vi "main.vi"(8 "error in (no error)":errorcluster, 11 "interface":T1) -> (0 "error out":errorcluster)   [LabVIEW 2015, in "lv-interface-sub-re.lvlib"]
uses:
  lv-interface-sub-re.lvlib
  lv-interface-sub-common/_controls/interface_selection.ctl
  private/_controls/hmi_references.ctl
  private/_controls/hmi_states.ctl
  private/_controls/event_common.ctl
  private/_controls/event_common_command.ctl
  private/_controls/event_interface.ctl
  private/_controls/event_interface_command.ctl
  private/_controls/menu_selection.ctl
  lv-interface-sub-common/lv-interface-sub-common.lvlib
panel:
  out "random_number":dbl
  out "source":string
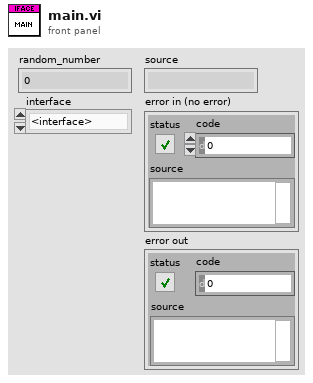
[diagram p1: front panel]
types:
  T1 = typedef "lv-interface-sub-common.lvlib/interface_selection.ctl" = enum16{"<interface>", "sub_interface_1", "sub_interface_2", "<null>"}
  T2 = typedef "lv-interface-sub-re.lvlib/hmi_references.ctl" = cluster{"vi_reference":refnum<vi>}
  T3 = typedef "lv-interface-sub-re.lvlib/event_interface.ctl" = cluster{"command":T4, "data":variant}
  T4 = typedef "lv-interface-sub-re.lvlib/event_interface_command.ctl" = enum16{"<event_interface_cmd>", "defer_panel_updates", "focus", "unfocus", "undefer_panel_updates", "<null>"}
  T5 = typedef "lv-interface-sub-re.lvlib/event_common.ctl" = cluster{"command":T6, "data":variant}
  T6 = typedef "lv-interface-sub-re.lvlib/event_common_command.ctl" = enum16{"<event_common_cmd>", "die", "<null>"}
  T7 = typedef "lv-interface-sub-re.lvlib/hmi_states.ctl" = enum16{"<hmi_states>", "initialize", "checkui", "updateui", "shutdown", "<null>"}
  T8 = typedef "lv-interface-sub-re.lvlib/menu_selection.ctl" = enum16{"<menu>", "file_exit", "help_about", "<null>"}
  T9 = typedef "interface_dom_nre.lvlib/interface_selection.ctl" = enum16{"<interface>", "sub_interface_1", "sub_interface_2", "<null>"}
  T10 = typedef "interface_sub_common.lvlib/event_to_sub_command.ctl" = enum16{"<to_sub_cmd>", "die", "focus", "unfocus", "<null>"}
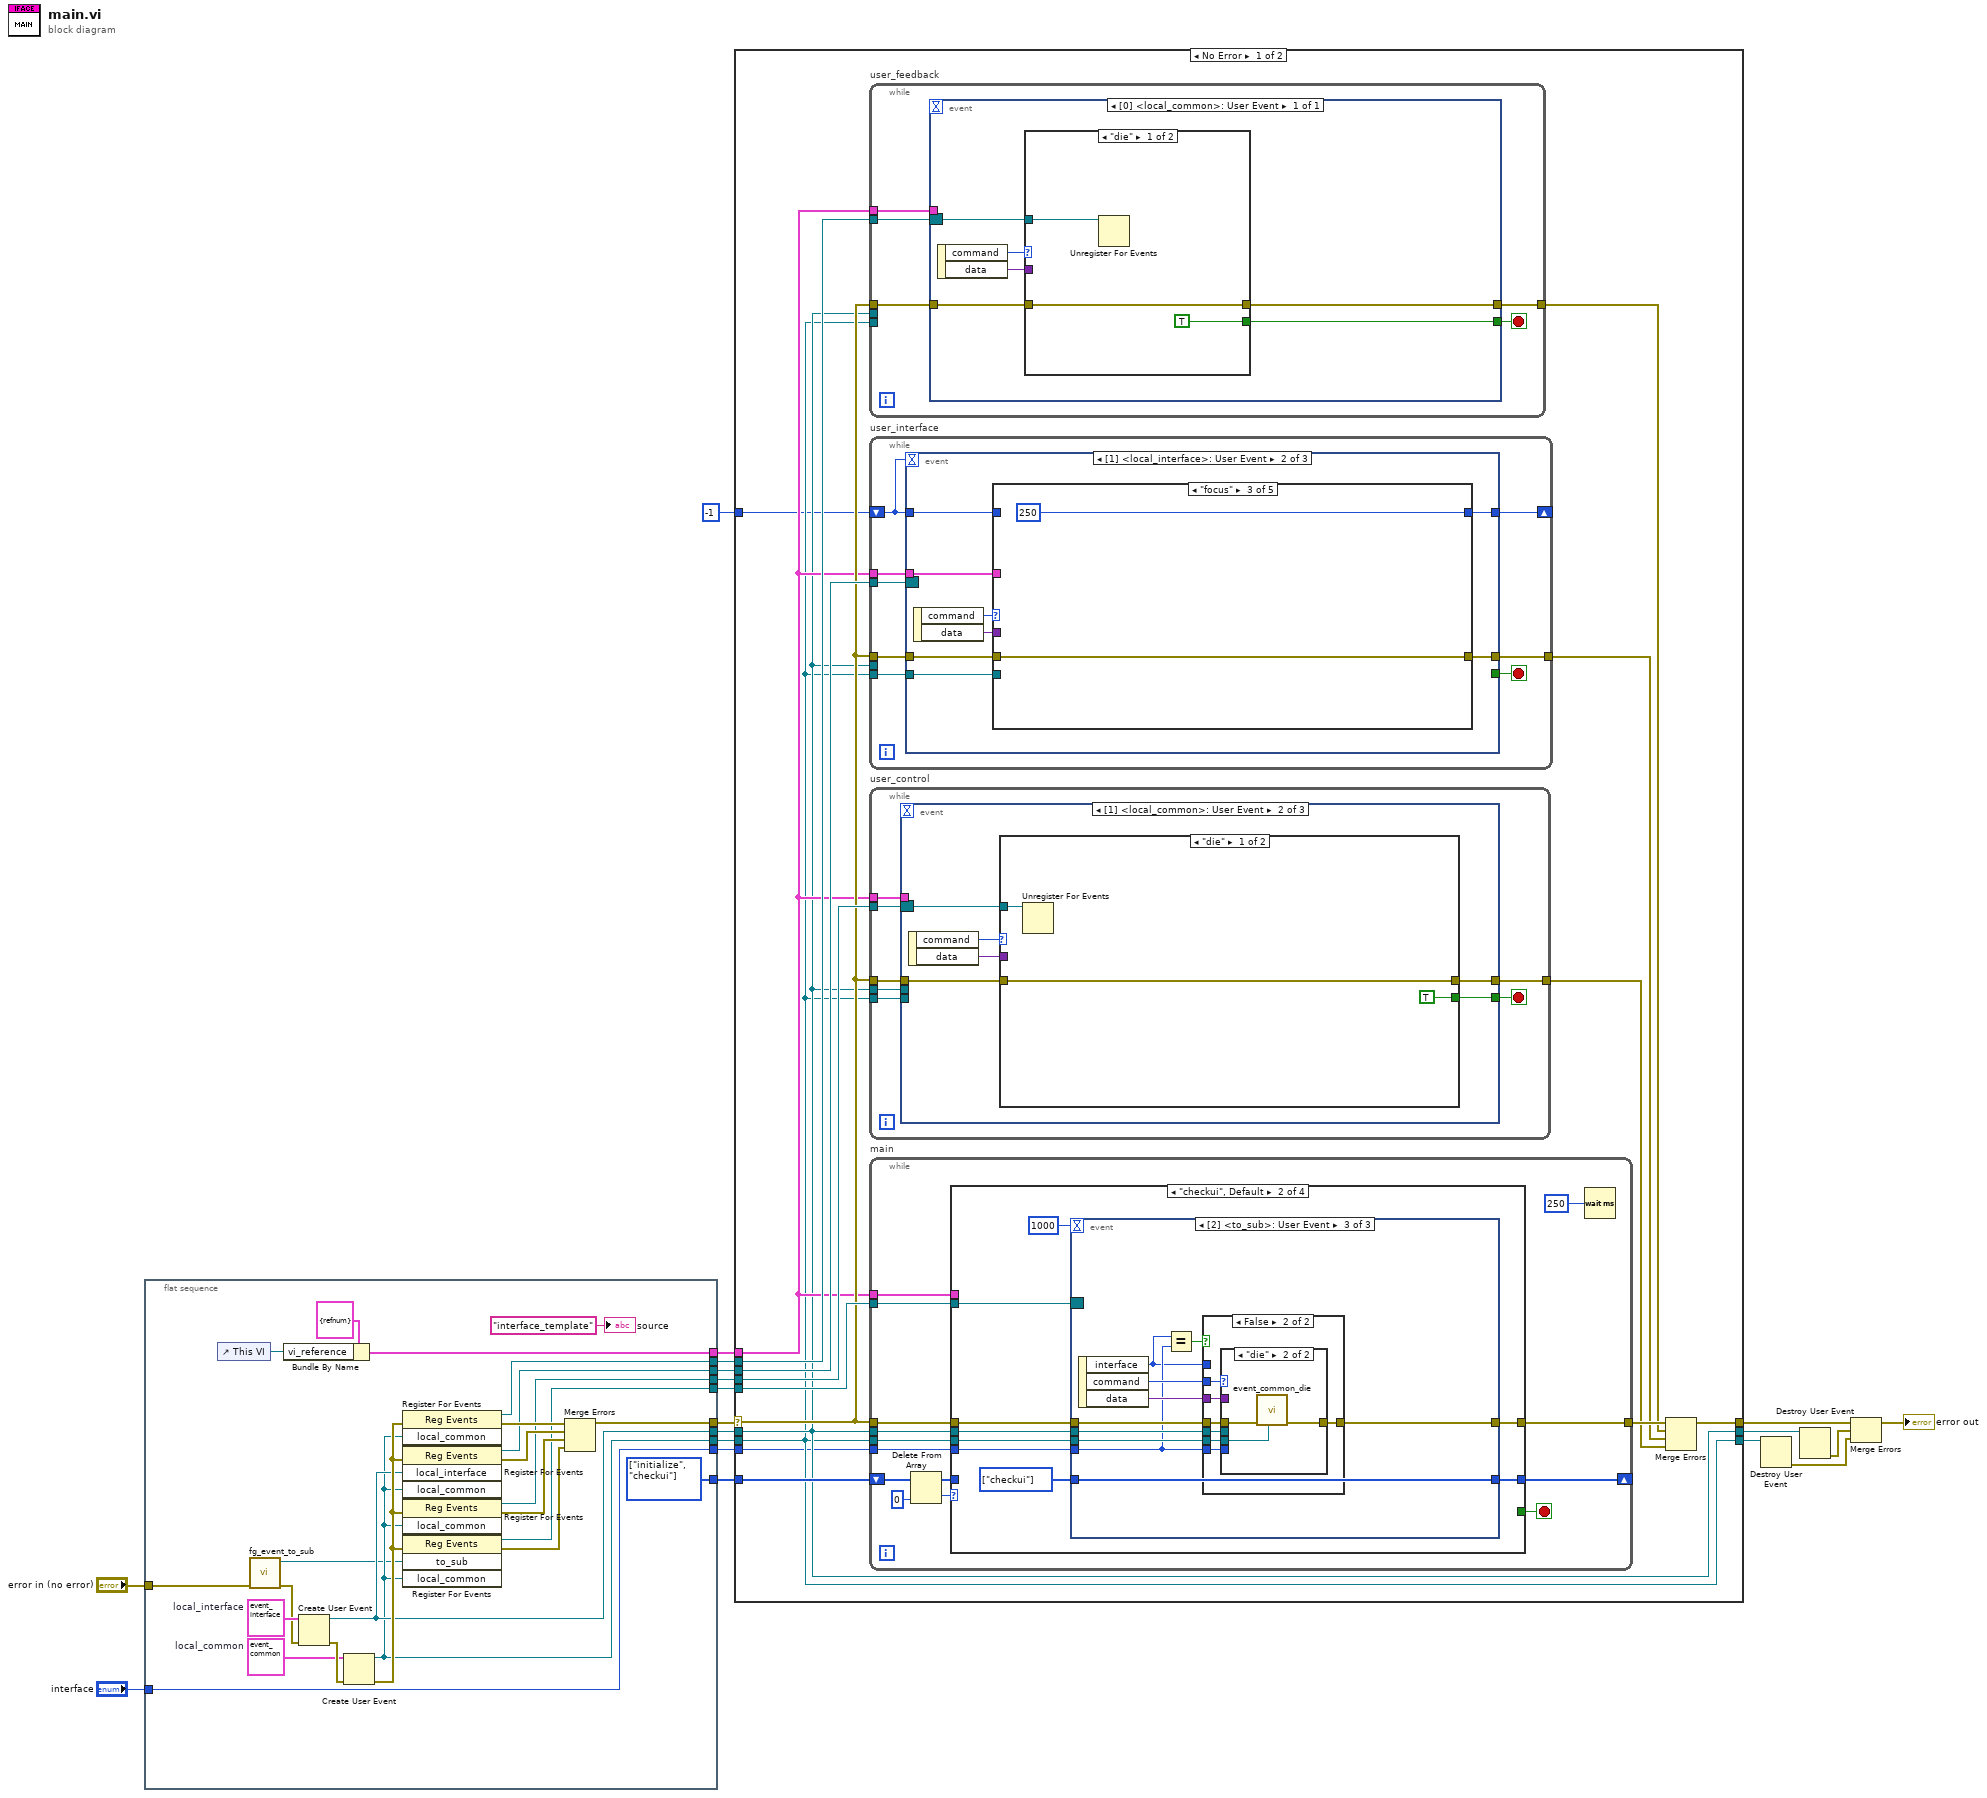
[diagram p0: block diagram]
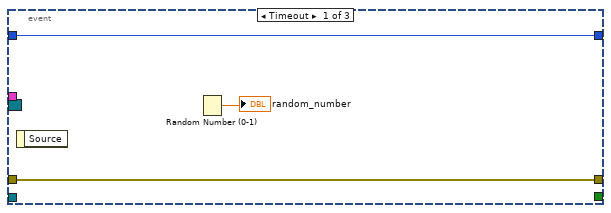
[diagram p3: hidden frame]
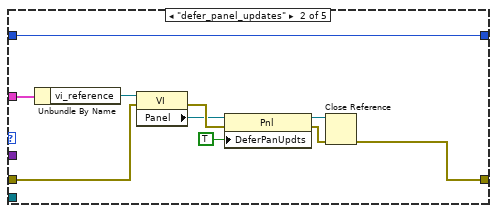
[diagram p5: hidden frame]
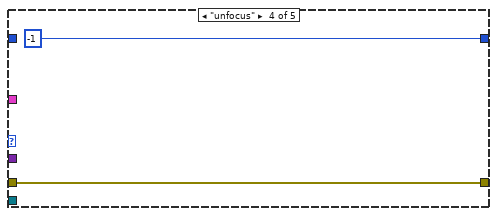
[diagram p6: hidden frame]
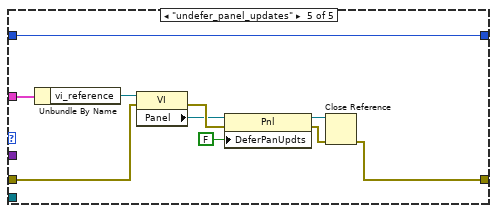
[diagram p7: hidden frame]
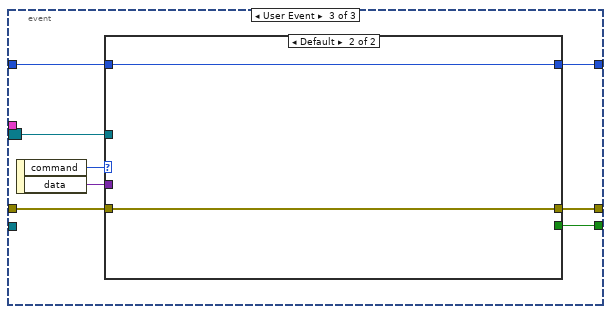
[diagram p8: hidden frame]
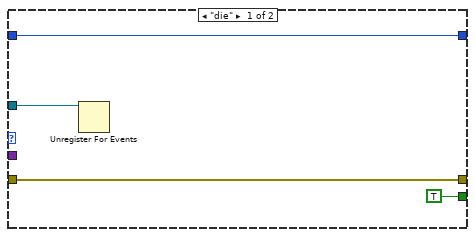
[diagram p9: hidden frame]
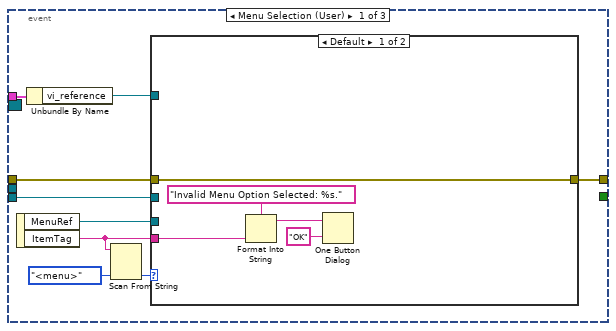
[diagram p10: hidden frame]
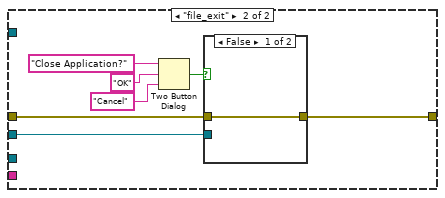
[diagram p11: hidden frame]
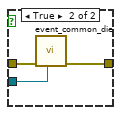
[diagram p12: hidden frame]
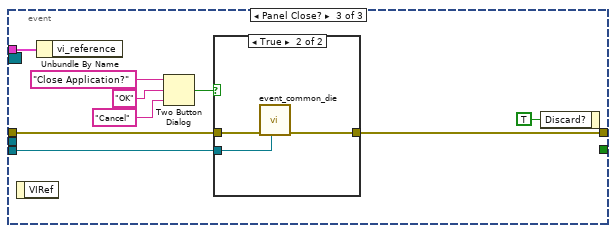
[diagram p14: hidden frame]
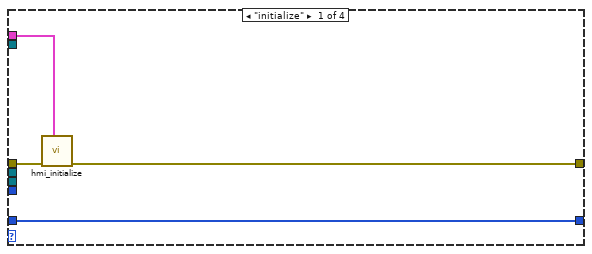
[diagram p16: hidden frame]
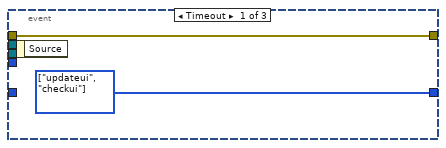
[diagram p17: hidden frame]
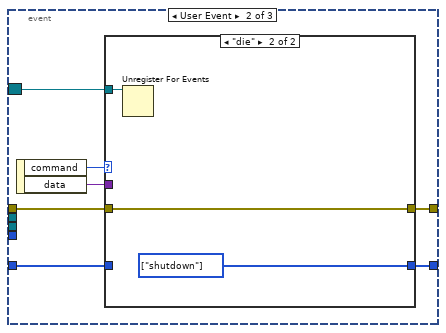
[diagram p18: hidden frame]
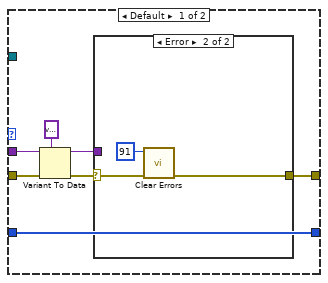
[diagram p19: hidden frame]
diagram:
  n1 = flat-sequence {
    tunnel: [w35] -> w19
    tunnel: [w34] -> w18
    tunnel: [w38] -> w17
    tunnel: "error in (no error)" -> [w22]
    tunnel: [w33] -> w15
    tunnel: [w32] -> w14
    tunnel: [w30] -> w13
    tunnel: [w24] -> w11
    tunnel: [w27] -> w12
    tunnel: [w25] -> w5
    tunnel: "interface" -> [w20]
    tunnel: [w20] -> w1
    frame #0 {
      w28 = T3 {"command"=enum."<event_interface_cmd>", "data"=variant}  # local_interface
      w29 = T5 {"command"=enum."<event_common_cmd>", "data"=variant}  # local_common
      w38 = T7[] [enum."initialize", enum."checkui"] items=["<hmi_states>", "initialize", "checkui", "updateui", "shutdown", "<null>"]
      n2 = control-ref of="This VI"() -> (w31:refnum<vi>)
      n3 = call "fg_event_to_sub.vi"("error in (no error)"=w22) -> ("error out"=w21:errorcluster, "to_sub"=w23:refnum<user-event>)  [unwired: 8 in, 1 out]
      n4 = Bundle By Name(cluster=T2 {"vi_reference"=refnum}, "vi_reference"=w31) -> (w30:T2)
      n5 = Create User Event(user event datatype=w28, error in=w21) -> (user event=w27:refnum<user-event>, error out=w42:errorcluster)
      n6 = Create User Event(user event datatype=w29, error in=w42) -> (user event=w24:refnum<user-event>, error out=w41:errorcluster)
      n7 = register-events(error in=w41, w24) -> (reference out=w25:refnum<event-registration>, error out=w43:errorcluster)  [unwired: 1 in]
      n8 = register-events(error in=w41, w27, w24) -> (reference out=w32:refnum<event-registration>, error out=w40:errorcluster)  [unwired: 1 in]
      n9 = register-events(error in=w41, w24) -> (reference out=w34:refnum<event-registration>, error out=w37:errorcluster)  [unwired: 1 in]
      n10 = register-events(error in=w41, w23, w24) -> (reference out=w33:refnum<event-registration>, error out=w36:errorcluster)  [unwired: 1 in]
      n11 = Merge Errors(w43, w40, w37, w36) -> (w35:errorcluster)
      "source" <- "interface_template" ("Source")
    }
  }
  n12 = case shown="No Error" w19 {
    selector: w19 -> [w50 w290]
    tunnel: w18 -> [w53 w286]
    tunnel: w17 -> [w55 _]
    tunnel: [w51 w290] -> w8
    tunnel: w15 -> [w54 w285]
    tunnel: w14 -> [w52 w287]
    tunnel: w13 -> [w49 _]
    tunnel: w12 -> [w48 w289]
    tunnel: w11 -> [w47 w288]
    tunnel: [w48 w289] -> w9
    tunnel: [w47 w288] -> w10
    tunnel: w5 -> [w59 w284]
    tunnel: -1 -> [w45 _]
    tunnel: w1 -> [w44 _]
    frame No Error {
      n13 = while "user_feedback" {
        tunnel: [w64] -> w46
        tunnel: w50 -> [w63]
        tunnel: w59 -> [w62]
        tunnel: w49 -> [w61]
        tunnel: w48 -> [_]
        tunnel: w47 -> [_]
        stop <- w60 stop-if-true
        n14 = event shown="[0] <local_common>: User Event" {
          selector: w62 -> [w70]
          dyn-events: _ -> [_]
          timeout: _ -> [_]
          tunnel: [w67] -> w64
          tunnel: w63 -> [w68]
          tunnel: w61 -> [_]
          tunnel: [w66] -> w60
          event User Event {
            n15 = event-data() -> ("command"=w69:T6, "data"=w65:variant)  [unwired: 1 in]
            n16 = case shown="\"die\"" w69 {
              tunnel: w68 -> [w72 w74]
              tunnel: [w72 w74] -> w67
              tunnel: [TRUE _] -> w66
              tunnel: w70 -> [w71 _]
              tunnel: w65 -> [_ _]
              frame "die" {
                n17 = Unregister For Events(event registration refnum=w71) -> ()  [unwired: 1 in, 1 out]
              }
              frame Default {
              }
            }
          }
        }
      }
      n18 = while "user_interface" {
        tunnel: w50 -> [w82]
        tunnel: [w80] -> w56
        tunnel: w52 -> [w79]
        tunnel: w48 -> [_]
        tunnel: w47 -> [w78]
        tunnel: w49 -> [w77]
        shift-right: [w76] -> _
        shift-left: w45 -> [w75]
        stop <- w81 stop-if-true
        n19 = event shown="[1] <local_interface>: User Event" {
          selector: w79 -> [_ _ w123]
          dyn-events: _ -> [_ _ _]
          timeout: w75 -> [_ _ _]
          tunnel: w82 -> [w83 w91 w126]
          tunnel: [w83 w90 w125] -> w80
          tunnel: [_ _ w124] -> w81
          tunnel: w78 -> [_ w89 _]
          tunnel: w77 -> [_ w88 _]
          tunnel: w75 -> [w85 w87 w121]
          tunnel: [w85 w86 w120] -> w76
          event Timeout {
            n20 = event-data() -> ()  [unwired: 1 in, 1 out]
            n21 = Random Number (0-1)() -> (number: 0 to 1=→"random_number":dbl)
          }
          event User Event {
            n22 = event-data() -> ("command"=w93:T4, "data"=w92:variant)  [unwired: 1 in]
            n23 = case shown="\"focus\"" w93 {
              tunnel: w91 -> [w94 w100 w106 w108 w114]
              tunnel: [w94 w99 w106 w108 w111] -> w90
              tunnel: w92 -> [_ _ _ _ _]
              tunnel: w89 -> [_ _ _ _ _]
              tunnel: w88 -> [_ w98 _ _ w113]
              tunnel: w87 -> [w95 w96 _ _ w110]
              tunnel: [w95 w96 250 -1 w110] -> w86
              frame Default {
              }
              frame "defer_panel_updates" {
                n24 = Unbundle By Name(w98) -> ("vi_reference"=w97:refnum<vi>)
                n25 = property class="VI"(reference=w97, error in=w100) -> (error out=w105:errorcluster, "Panel"=w101:refnum<vi>)  [unwired: 1 out]
                n26 = property class="Pnl"(reference=w101, error in=w105, "DeferPanUpdts"=TRUE ("Defer Panel Updates")) -> (reference out=w103:refnum<vi>, error out=w102:errorcluster)
                n27 = Close Reference(reference=w103, error in (no error)=w102) -> (error out=w99:errorcluster)
              }
              frame "focus" {
              }
              frame "unfocus" {
              }
              frame "undefer_panel_updates" {
                n28 = Unbundle By Name(w113) -> ("vi_reference"=w112:refnum<vi>)
                n29 = property class="VI"(reference=w112, error in=w114) -> (error out=w119:errorcluster, "Panel"=w115:refnum<vi>)  [unwired: 1 out]
                n30 = property class="Pnl"(reference=w115, error in=w119, "DeferPanUpdts"=FALSE ("Defer Panel Updates")) -> (reference out=w117:refnum<vi>, error out=w116:errorcluster)
                n31 = Close Reference(reference=w117, error in (no error)=w116) -> (error out=w111:errorcluster)
              }
            }
          }
          event User Event {
            n32 = event-data() -> ("command"=w127:T6, "data"=w122:variant)  [unwired: 1 in]
            n33 = case shown="Default" w127 {
              tunnel: w126 -> [w130 w133]
              tunnel: [w130 w133] -> w125
              tunnel: [TRUE _] -> w124
              tunnel: w123 -> [w129 _]
              tunnel: w122 -> [_ _]
              tunnel: w121 -> [w128 w132]
              tunnel: [w128 w132] -> w120
              frame "die" {
                n34 = Unregister For Events(event registration refnum=w129) -> ()  [unwired: 1 in, 1 out]
              }
              frame Default {
              }
            }
          }
        }
      }
      n35 = while "user_control" {
        tunnel: w50 -> [w140]
        tunnel: [w138] -> w57
        tunnel: w53 -> [w137]
        tunnel: w48 -> [w135]
        tunnel: w47 -> [w134]
        tunnel: w49 -> [w136]
        stop <- w139 stop-if-true
        n36 = event shown="[1] <local_common>: User Event" {
          selector: w137 -> [_ w166 _]
          dyn-events: _ -> [_ _ _]
          timeout: _ -> [_ _ _]
          tunnel: w140 -> [w146 w170 w176]
          tunnel: [w144 w169 w183] -> w138
          tunnel: [_ w168 _] -> w139
          tunnel: w136 -> [w143 _ w182]
          tunnel: w135 -> [_ _ _]
          tunnel: w134 -> [w141 _ w181]
          event Menu Selection (User) {
            n37 = event-data() -> ("MenuRef"=w147:refnum<k9>, "ItemTag"=w145:string)  [unwired: 1 in]
            n38 = Unbundle By Name(w143) -> ("vi_reference"=w142:refnum<vi>)
            n39 = Scan From String(input string=w145, default 1=menu_selection."<menu>" ("menu_selection")) -> (output 1=w148:T8)  [unwired: 3 in, 3 out]
            n40 = case shown="Default" w148 {
              tunnel: w147 -> [_ _]
              tunnel: w146 -> [w150 w155]
              tunnel: w145 -> [w154 _]
              tunnel: [w150 w161] -> w144
              tunnel: w142 -> [_ _]
              tunnel: w141 -> [_ w160]
              frame Default {
                n41 = Format Into String(format string="Invalid Menu Option Selected: %s.", w154) -> (resulting string=w152:string)  [unwired: 2 in, 1 out]
                n42 = One Button Dialog(message=w152, button name ("OK")="OK" ("boolean_text_1")) -> ()  [unwired: 1 out]
              }
              frame "file_exit" {
                n43 = Two Button Dialog(message="Close Application?" ("dialog_text"), 1:"Cancel" ("boolean_text_1"), 2:"OK" ("boolean_text_1")) -> (T button?=w156:bool)
                n44 = case shown="False" w156 {
                  tunnel: w155 -> [w162 w165]
                  tunnel: [w162 w164] -> w161
                  tunnel: w160 -> [_ w163]
                  frame False {
                  }
                  frame True {
                    n45 = call "event_common_die.vi"("local_common"=w163, "error in (no error)"=w165) -> ("error out"=w164:errorcluster)  [unwired: 9 in]
                  }
                }
              }
            }
          }
          event User Event {
            n46 = event-data() -> ("command"=w171:T6, "data"=w167:variant)  [unwired: 1 in]
            n47 = case shown="\"die\"" w171 {
              tunnel: w170 -> [w172 w175]
              tunnel: [w172 w175] -> w169
              tunnel: [TRUE _] -> w168
              tunnel: w167 -> [_ _]
              tunnel: w166 -> [w173 _]
              frame "die" {
                n48 = Unregister For Events(event registration refnum=w173) -> ()  [unwired: 1 in, 1 out]
              }
              frame Default {
              }
            }
          }
          event Panel Close? {
            n49 = event-data() -> ()  [unwired: 1 in, 1 out]
            n50 = Unbundle By Name(w182) -> ()  [unwired: 1 out]
            n51 = Two Button Dialog(message="Close Application?" ("dialog_text"), 1:"Cancel" ("boolean_text_1"), 2:"OK" ("boolean_text_1")) -> (T button?=w177:bool)
            n52 = case shown="True" w177 {
              tunnel: w176 -> [w185 w188]
              tunnel: [w185 w187] -> w183
              tunnel: w181 -> [_ w186]
              frame False {
              }
              frame True {
                n53 = call "event_common_die.vi"("local_common"=w186, "error in (no error)"=w188) -> ("error out"=w187:errorcluster)  [unwired: 9 in]
              }
            }
            n54 = event-data("Discard?"=TRUE) -> ()  [unwired: 1 in, 1 out]
          }
        }
      }
      n55 = while "main" {
        shift-right: [w194] -> _
        shift-left: w55 -> [w201]
        tunnel: w54 -> [w195]
        tunnel: w50 -> [w197]
        tunnel: [w193] -> w58
        tunnel: w49 -> [w192]
        tunnel: w47 -> [w191]
        tunnel: w48 -> [w190]
        tunnel: w44 -> [w189]
        stop <- w196 stop-if-true
        n56 = Delete From Array(array=w201, index=0) -> (deleted portion=w199:T7, array with subset deleted=w198:T7[])  [unwired: 1 in]
        n57 = case shown="\"checkui\", Default" w199 {
          tunnel: w198 -> [w206 _ w278 _]
          tunnel: w197 -> [w205 w214 w277 w282]
          tunnel: [_ _ _ TRUE] -> w196
          tunnel: [w203 w213 w277 w281] -> w193
          tunnel: [w206 w212 w278 w280] -> w194
          tunnel: w195 -> [_ w210 _ _]
          tunnel: w192 -> [w204 _ _ w279]
          tunnel: w191 -> [_ w208 _ _]
          tunnel: w190 -> [_ w209 _ _]
          tunnel: w189 -> [_ w207 _ _]
          frame "initialize" {
            n58 = call "hmi_initialize.vi"("hmi_references"=w204, "error in (no error)"=w205) -> ("error out"=w203:errorcluster)  [unwired: 9 in]
          }
          frame "checkui", Default {
            w211 = T7[] [enum."checkui"] items=["<hmi_states>", "initialize", "checkui", "updateui", "shutdown", "<null>"]
            n59 = event shown="[2] <to_sub>: User Event" {
              selector: w210 -> [_ w218 _]
              dyn-events: _ -> [_ _ _]
              timeout: 1000 -> [_ _ _]
              tunnel: w214 -> [w217 w222 w246]
              tunnel: [w217 w219 w245] -> w213
              tunnel: [w216 w220 w242] -> w212
              tunnel: w211 -> [_ w221 w242]
              tunnel: w209 -> [_ _ w244]
              tunnel: w208 -> [_ _ w243]
              tunnel: w207 -> [_ _ w241]
              event Timeout {
                w216 = T7[] [enum."updateui", enum."checkui"] items=["<hmi_states>", "initialize", "checkui", "updateui", "shutdown", "<null>"]
                n60 = event-data() -> ()  [unwired: 1 in, 1 out]
              }
              event User Event {
                n61 = event-data() -> ("command"=w224:T6, "data"=w223:variant)  [unwired: 1 in]
                n62 = case shown="\"die\"" w224 {
                  tunnel: [w231 w238] -> w220
                  tunnel: w221 -> [w231 _]
                  tunnel: w222 -> [w229 w237]
                  tunnel: [w225 w237] -> w219
                  tunnel: w223 -> [w230 _]
                  tunnel: w218 -> [_ w236]
                  frame Default {
                    n63 = Variant To Data(error in=w229, type=variant, Variant=w230) -> (data=w226:variant, error out=w228:errorcluster)
                    n64 = case shown="Error" w228 {
                      selector: w228 -> [w232 w235]
                      tunnel: w226 -> [_ _]
                      tunnel: [w232 w234] -> w225
                      frame No Error {
                      }
                      frame Error {
                        n65 = call <vilib>:"Clear Errors.vi"("error in (no error)"=w235, "specific error code to clear (0: all)"=91) -> ("error out"=w234:errorcluster)  [unwired: 4 in, 1 out]
                      }
                    }
                  }
                  frame "die" {
                    w238 = T7[] [enum."shutdown"] items=["<hmi_states>", "initialize", "checkui", "updateui", "shutdown", "<null>"]
                    n66 = Unregister For Events(event registration refnum=w236) -> ()  [unwired: 1 in, 1 out]
                  }
                }
              }
              event User Event {
                n67 = event-data() -> ("interface"=w240:T9, "command"=w248:T10, "data"=w247:variant)  [unwired: 1 in]
                n68 = Equal?(x=w240, y=w241) -> (x = y?=w239:bool)
                n69 = case shown="False" w239 {
                  tunnel: w248 -> [w255 w272]
                  tunnel: w247 -> [w254 w271]
                  tunnel: w246 -> [w253 w270]
                  tunnel: [w252 w269] -> w245
                  tunnel: w240 -> [_ _]
                  tunnel: w244 -> [w251 w268]
                  tunnel: w243 -> [w250 w267]
                  tunnel: w241 -> [w249 w266]
                  frame True {
                    n70 = case shown="\"die\"" w255 {
                      tunnel: w253 -> [w256 w258 w262 w264]
                      tunnel: [w256 w257 w260 w263] -> w252
                      tunnel: w254 -> [_ _ _ _]
                      tunnel: w251 -> [_ w259 w261 _]
                      tunnel: w250 -> [_ _ _ w265]
                      tunnel: w249 -> [_ _ _ _]
                      frame Default {
                      }
                      frame "focus" {
                        n71 = call "event_interface_focus.vi"("event_interface"=w259, "error in (no error)"=w258) -> ("error out"=w257:errorcluster)  [unwired: 9 in]
                      }
                      frame "unfocus" {
                        n72 = call "event_interface_unfocus.vi"("event_interface"=w261, "error in (no error)"=w262) -> ("error out"=w260:errorcluster)  [unwired: 9 in]
                      }
                      frame "die" {
                        n73 = call "event_common_die.vi"("local_common"=w265, "error in (no error)"=w264) -> ("error out"=w263:errorcluster)  [unwired: 9 in]
                      }
                    }
                  }
                  frame False {
                    n74 = case shown="\"die\"" w272 {
                      tunnel: w270 -> [w273 w275]
                      tunnel: [w273 w274] -> w269
                      tunnel: w271 -> [_ _]
                      tunnel: w268 -> [_ _]
                      tunnel: w267 -> [_ w276]
                      tunnel: w266 -> [_ _]
                      frame Default {
                      }
                      frame "die" {
                        n75 = call "event_common_die.vi"("local_common"=w276, "error in (no error)"=w275) -> ("error out"=w274:errorcluster)  [unwired: 9 in]
                      }
                    }
                  }
                }
              }
            }
          }
          frame "updateui" {
          }
          frame "shutdown" {
            w280 = T7[] [enum."shutdown"] items=["<hmi_states>", "initialize", "checkui", "updateui", "shutdown", "<null>"]
            n76 = call "hmi_shutdown.vi"("hmi_references"=w279, "error in (no error)"=w282) -> ("error out"=w281:errorcluster)  [unwired: 9 in]
          }
        }
        n77 = Wait (ms)(milliseconds to wait=u32 250) -> ()  [unwired: 1 out]
      }
      n78 = Merge Errors(w58, w46, w56, w57) -> (w51:errorcluster)
    }
    frame Error {
      n79 = Unregister For Events(event registration refnum=w285) -> ()  [unwired: 1 in, 1 out]
      n80 = Unregister For Events(event registration refnum=w286) -> ()  [unwired: 1 in, 1 out]
      n81 = Unregister For Events(event registration refnum=w287) -> ()  [unwired: 1 in, 1 out]
      n82 = Unregister For Events(event registration refnum=w284) -> ()  [unwired: 1 in, 1 out]
    }
  }
  n83 = Destroy User Event(user event=w10) -> (error out=w6:errorcluster)  [unwired: 1 in]
  n84 = Destroy User Event(user event=w9) -> (error out=w7:errorcluster)  [unwired: 1 in]
  n85 = Merge Errors(w8, w7, w6) -> (→"error out":errorcluster)
